vi "Sine Generator (FPGA).vi"() -> ()   [LabVIEW 2012]
doc: "This VI uses the Sine Wave Generator function to create sine wave signals for the outputs. The frequency, phase, offset, and amplitude of the sinewaves can be programmatically changed from the host VI.s"
panel:
  out "Output 1":i16
  out "Output 0":i16
  in  "Initialize":bool
  in  "Sinewave Props 1":T1={"Frequency (periods/tick)"=0.0, "Phase offset (periods)"=0.0, "Scale factor"=0.999969482421875, "Amplitude offset"=0.0}
  in  "Sinewave Props 0":T1={"Frequency (periods/tick)"=0.0, "Phase offset (periods)"=0.0, "Scale factor"=0.999969482421875, "Amplitude offset"=0.0}
  out "Sampling rate achieved?":bool
  out "Actual loop rate":u32
  in  "Stop":bool
  in  "Desired loop rate (ticks)":u32=2666666 caption="Update Interval (Ticks)"
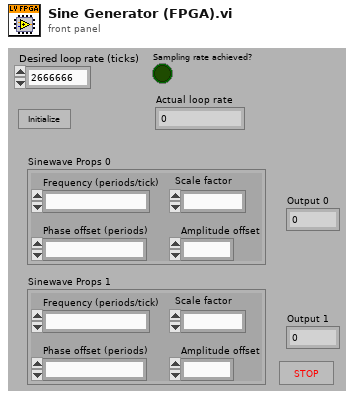
[diagram p1: front panel]
types:
  T1 = cluster{"Frequency (periods/tick)":fxp<+,32,0>, "Phase offset (periods)":fxp<+,32,0>, "Scale factor":fxp<+/-,16,1>, "Amplitude offset":fxp<+/-,16,16>}
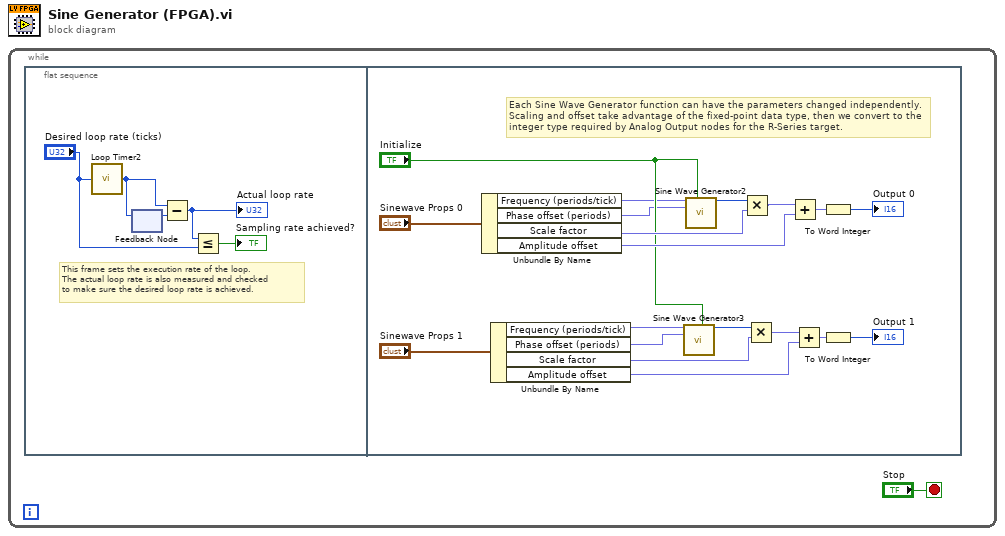
[diagram p0: block diagram]
diagram:
  n1 = while {
    stop <- "Stop" stop-if-true
    n2 = flat-sequence {
      frame #0 {
        # "This frame sets the execution rate of the loop.\nThe actual loop rate is also measured and checked\nto make sure the desired loop rate is achieved."
        n3 = call "Loop Timer2"("Count(Ticks)"="Desired loop rate (ticks)") -> ("Tick Count(Ticks)"=w2:u32)
        n4 = feedback-in #1(w2) -> ()
        n5 = feedback #1() -> (w4:u32)  [unwired: 1 out]
        n6 = Subtract(x=w2, y=w4) -> (x-y=w6:u32)
        "Actual loop rate" <- w6
        n7 = Less Or Equal?(x=w6, y="Desired loop rate (ticks)") -> (x <= y?=→"Sampling rate achieved?":bool)
      }
      frame #1 {
        # "Each Sine Wave Generator function can have the parameters changed independently.\nScaling and offset take advantage of the fixed-point data type, then we convert to the\ninteger type required by Analog Output nodes for the R-Series target."
        n8 = Unbundle By Name("Sinewave Props 0") -> ("Frequency (periods/tick)"=w19:fxp<+,32,0>, "Phase offset (periods)"=w18:fxp<+,32,0>, "Scale factor"=w24:fxp<+/-,16,1>, "Amplitude offset"=w23:fxp<+/-,16,16>)
        n9 = Unbundle By Name("Sinewave Props 1") -> ("Frequency (periods/tick)"=w14:fxp<+,32,0>, "Phase offset (periods)"=w13:fxp<+,32,0>, "Scale factor"=w12:fxp<+/-,16,1>, "Amplitude offset"=w10:fxp<+/-,16,16>)
        n10 = call "Sine Wave Generator3"("frequency (periods/tick)"=w14, "reset"="Initialize", "phase offset (periods)"=w13) -> ("sine out"=w11:i16)  [unwired: 12 in]
        n11 = call "Sine Wave Generator2"("frequency (periods/tick)"=w19, "reset"="Initialize", "phase offset (periods)"=w18) -> ("sine out"=w21:i16)  [unwired: 12 in]
        n12 = Multiply(x=w21, y=w24) -> (x*y=w16:fxp<+/-,32,17>)
        n13 = Multiply(x=w11, y=w12) -> (x*y=w15:fxp<+/-,32,17>)
        n14 = Add(x=w16, y=w23) -> (x+y=w22:fxp<+/-,16,16>)
        n15 = Add(x=w15, y=w10) -> (x+y=w9:fxp<+/-,16,16>)
        n16 = To Word Integer(number=w22) -> (16bit integer=→"Output 0":i16)
        n17 = To Word Integer(number=w9) -> (16bit integer=→"Output 1":i16)
      }
    }
  }
